vi "rethinkdb_tcp_parse_messages.vi"(11 "data in":string) -> (2 "unterminated?":bool, 3 "messages":string[](array[string]))   [LabVIEW 2017]
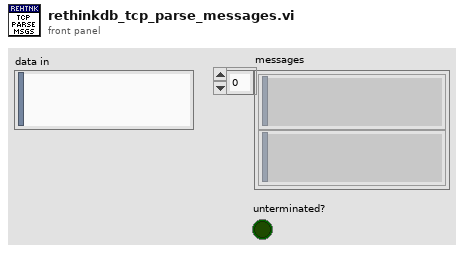
[diagram p1: front panel]
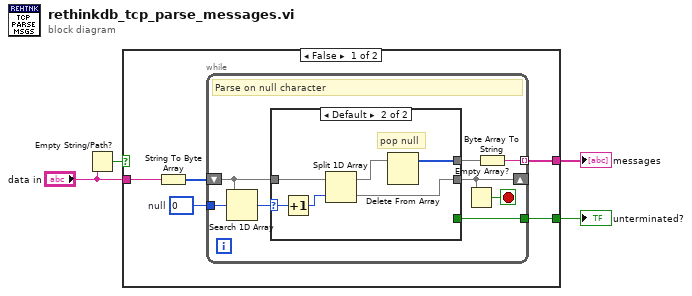
[diagram p0: block diagram]
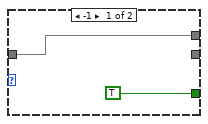
[diagram p2: hidden frame]
diagram:
  n1 = Empty String/Path?(string/path="data in") -> (empty?=w1:bool)
  n2 = case shown="False" w1 {
    tunnel: "data in" -> [w9 _]
    tunnel: [w6 _] -> w4
    tunnel: [w5 _] -> w3
    frame False {
      w7 = u8 0  # null
      n3 = String To Byte Array(string=w9) -> (unsigned byte array=w8:u8[])
      n4 = while {
        shift-right: [w14] -> _
        shift-left: w8 -> [w16]
        tunnel: w7 -> [w17]
        tunnel: [w11] -> w6 mode=indexing
        tunnel: [w10] -> w5
        stop <- w13 stop-if-true
        # "Parse on null character"
        n5 = Search 1D Array(1D array=w16, element=w17) -> (index of element=w15:i32)  [unwired: 1 in]
        n6 = case shown="Default" w15 {
          selector: w15 -> [_ w24]
          tunnel: w16 -> [w19 w25]
          tunnel: [_ w22] -> w14
          tunnel: [w19 w20] -> w12
          tunnel: [TRUE _] -> w10
          frame -1 {
          }
          frame Default {
            # "pop null"
            n7 = Increment(x=w24) -> (x+1=w23:i32)
            n8 = Split 1D Array(array=w25, index=w23) -> (first subarray=w21:u8[], second subarray=w22:u8[])
            n9 = Delete From Array(array=w21) -> (array with subset deleted=w20:u8[])  [unwired: 2 in, 1 out]
          }
        }
        n10 = Empty Array?(array=w14) -> (empty?=w13:bool)
        n11 = Byte Array To String(unsigned byte array=w12) -> (string=w11:string)
      }
    }
    frame True {
    }
  }
  "messages" <- w4
  "unterminated?" <- w3
